vi "Solar Panel.vi"() -> ()   [LabVIEW 2013]
panel:
  out "Light ON Right?":bool
  out "Light ON Left?":bool
  out "Light ON?":bool
  in  "STATE":T1(ring)
  out "Right Photocell":dbl(slide) scale=0.0..1000.0
  out "Left Photocell":dbl(slide) scale=0.0..1000.0
  in  "Stop Button":bool
  out "Panel Up Limit Switch":bool
  out "Panel Down Limit Switch":bool
  out "Right Rotation Limit Switch":bool
  out "Left Rotation Limit Switch":bool
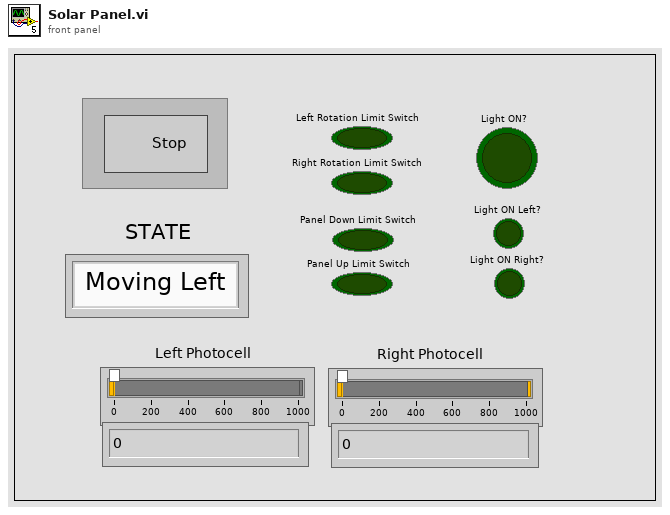
[diagram p1: front panel]
types:
  T1 = enum16{"Moving Left", "Moving Right", "Stopped", "Start Position"}
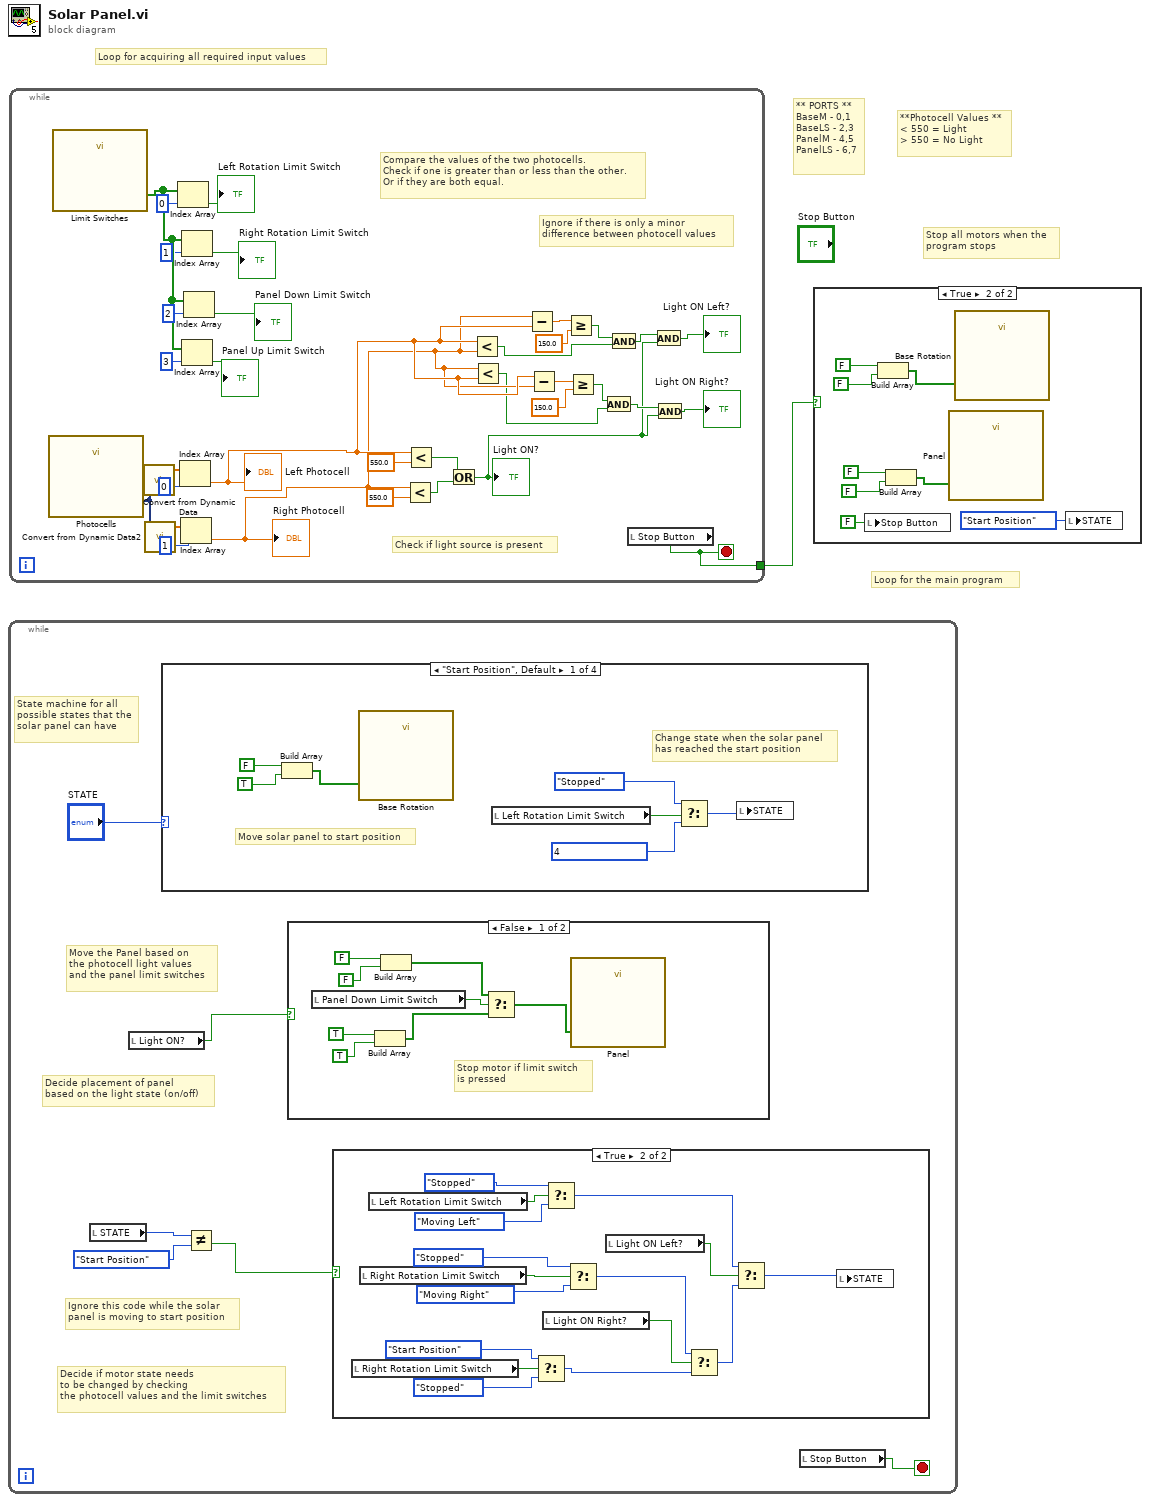
[diagram p0: block diagram]
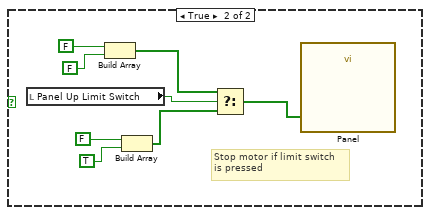
[diagram p4: hidden frame]
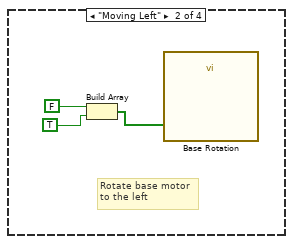
[diagram p5: hidden frame]
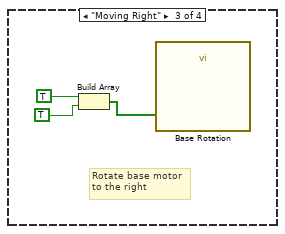
[diagram p6: hidden frame]
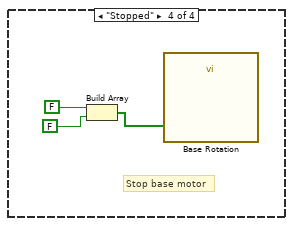
[diagram p7: hidden frame]
diagram:
  # "Stop all motors when the\nprogram stops"
  # "Loop for the main program"
  # "**Photocell Values **\n< 550 = Light\n> 550 = No Light"
  # "Loop for acquiring all required input values"
  # "** PORTS **\nBaseM - 0,1\nBaseLS - 2,3\nPanelM - 4,5\nPanelLS - 6,7"
  n1 = while {
    stop <- w2 stop-if-true
    # "Ignore this code while the solar\npanel is moving to start position"
    # "Decide if motor state needs\nto be changed by checking\nthe photocell values and the limit switches"
    # "State machine for all\npossible states that the\nsolar panel can have"
    # "Decide placement of panel\nbased on the light state (on/off)"
    # "Move the Panel based on\nthe photocell light values\nand the panel limit switches"
    n2 = local read "STATE"() -> (w5:T1)
    n3 = local read "Light ON?"() -> (w6:bool)
    n4 = case shown="\"Start Position\", Default" "STATE" {
      frame "Start Position", Default {
        # "Move solar panel to start position"
        # "Change state when the solar panel\nhas reached the start position"
        n5 = Build Array(FALSE, TRUE) -> (w44:bool[])
        n6 = call "Base Rotation"("data"=w44) -> ()  [unwired: 17 in, 2 out]
        n7 = local read "Left Rotation Limit Switch"() -> (w43:bool)
        n8 = Select(t=T1."Stopped" ("State"), s=w43, f=T1 4 ("State")) -> (s? t:f=w40:T1)
        n9 = local write "STATE"(w40) -> ()
      }
      frame "Moving Left" {
        # "Rotate base motor\nto the left"
        n10 = Build Array(FALSE, TRUE) -> (w47:bool[])
        n11 = call "Base Rotation"("data"=w47) -> ()  [unwired: 17 in, 2 out]
      }
      frame "Moving Right" {
        # "Rotate base motor\nto the right"
        n12 = Build Array(TRUE, TRUE) -> (w50:bool[])
        n13 = call "Base Rotation"("data"=w50) -> ()  [unwired: 17 in, 2 out]
      }
      frame "Stopped" {
        # "Stop base motor"
        n14 = Build Array(FALSE, FALSE) -> (w53:bool[])
        n15 = call "Base Rotation"("data"=w53) -> ()  [unwired: 17 in, 2 out]
      }
    }
    n16 = Not Equal?(x=w5, y=T1."Start Position") -> (x != y?=w3:bool)
    n17 = case shown="False" w6 {
      frame False {
        # "Stop motor if limit switch\nis pressed"
        n18 = local read "Panel Down Limit Switch"() -> (w24:bool)
        n19 = Build Array(TRUE, TRUE) -> (w25:bool[])
        n20 = Build Array(FALSE, FALSE) -> (w28:bool[])
        n21 = Select(t=w28, s=w24, f=w25) -> (s? t:f=w29:bool[])
        n22 = call "Panel"("data"=w29) -> ()  [unwired: 17 in, 2 out]
      }
      frame True {
        # "Stop motor if limit switch\nis pressed"
        n23 = local read "Panel Up Limit Switch"() -> (w32:bool)
        n24 = Build Array(FALSE, FALSE) -> (w39:bool[])
        n25 = Build Array(FALSE, TRUE) -> (w33:bool[])
        n26 = Select(t=w39, s=w32, f=w33) -> (s? t:f=w34:bool[])
        n27 = call "Panel"("data"=w34) -> ()  [unwired: 17 in, 2 out]
      }
    }
    n28 = case shown="True" w3 {
      frame False {
      }
      frame True {
        n29 = local read "Right Rotation Limit Switch"() -> (w11:bool)
        n30 = local read "Right Rotation Limit Switch"() -> (w17:bool)
        n31 = local read "Left Rotation Limit Switch"() -> (w22:bool)
        n32 = Select(t=T1."Start Position" ("State"), s=w11, f=T1."Stopped" ("State")) -> (s? t:f=w9:T1)
        n33 = local read "Light ON Right?"() -> (w18:bool)
        n34 = Select(t=T1."Stopped" ("State"), s=w22, f=T1."Moving Left" ("State")) -> (s? t:f=w20:T1)
        n35 = Select(t=T1."Stopped" ("State"), s=w17, f=T1."Moving Right" ("State")) -> (s? t:f=w14:T1)
        n36 = local read "Light ON Left?"() -> (w12:bool)
        n37 = Select(t=w14, s=w18, f=w9) -> (s? t:f=w13:T1)
        n38 = Select(t=w20, s=w12, f=w13) -> (s? t:f=w19:T1)
        n39 = local write "STATE"(w19) -> ()
      }
    }
    n40 = local read "Stop Button"() -> (w2:bool)
  }
  n41 = while {
    tunnel: [w71] -> w1
    stop <- w71 stop-if-true
    # "Ignore if there is only a minor\ndifference between photocell values"
    # "Compare the values of the two photocells.\nCheck if one is greater than or less than the other.\nOr if they are both equal."
    # "Check if light source is present"
    n42 = call "Photocells"() -> ("data"=w79:dynamicdata)  [unwired: 17 in, 2 out]
    n43 = call "Limit Switches"() -> ("data"=w87:bool[])  [unwired: 17 in, 2 out]
    n44 = call "Convert from Dynamic Data"("Dynamic Data Type"=w79) -> ("Array"=w80:dbl[])  [unwired: 3 in]
    n45 = call "Convert from Dynamic Data2"("Dynamic Data Type"=w79) -> ("Array"=w78:dbl[])  [unwired: 3 in]
    n46 = Index Array(array=w87, index=0) -> (element=→"Left Rotation Limit Switch":bool)
    n47 = Index Array(array=w80, index=0) -> (element=w65:dbl)
    "Left Photocell" <- w65
    n48 = Index Array(array=w78, index=1) -> (element=w64:dbl)
    "Right Photocell" <- w64
    n49 = Index Array(array=w87, index=1) -> (element=→"Right Rotation Limit Switch":bool)
    n50 = Index Array(array=w87, index=3) -> (element=→"Panel Up Limit Switch":bool)
    n51 = Index Array(array=w87, index=2) -> (element=→"Panel Down Limit Switch":bool)
    n52 = Less?(x=w64, y=550.0) -> (x < y?=w72:bool)
    n53 = Less?(x=w65, y=550.0) -> (x < y?=w73:bool)
    n54 = Or(x=w73, y=w72) -> (x .or. y?=w56:bool)
    "Light ON?" <- w56
    n55 = Less?(x=w65, y=w64) -> (x < y?=w67:bool)
    n56 = Less?(x=w64, y=w65) -> (x < y?=w63:bool)
    n57 = Subtract(x=w64, y=w65) -> (x-y=w69:dbl)
    n58 = Subtract(x=w65, y=w64) -> (x-y=w61:dbl)
    n59 = Greater Or Equal?(x=w69, y=150.0) -> (x >= y?=w70:bool)
    n60 = Greater Or Equal?(x=w61, y=150.0) -> (x >= y?=w66:bool)
    n61 = And(x=w66, y=w63) -> (x .and. y?=w59:bool)
    n62 = And(x=w70, y=w67) -> (x .and. y?=w60:bool)
    n63 = local read "Stop Button"() -> (w71:bool)
    n64 = And(x=w60, y=w56) -> (x .and. y?=→"Light ON Left?":bool)
    n65 = And(x=w59, y=w56) -> (x .and. y?=→"Light ON Right?":bool)
  }
  n66 = case shown="True" w1 {
    frame False {
    }
    frame True {
      n67 = local write "Stop Button"(FALSE ("Stop Button")) -> ()
      n68 = Build Array(FALSE, FALSE) -> (w95:bool[])
      n69 = Build Array(FALSE, FALSE) -> (w92:bool[])
      n70 = call "Panel"("data"=w92) -> ()  [unwired: 17 in, 2 out]
      n71 = call "Base Rotation"("data"=w95) -> ()  [unwired: 17 in, 2 out]
      n72 = local write "STATE"(T1."Start Position" ("STATE")) -> ()
    }
  }
